vi "Dashboard Main.vi"() -> ()   [LabVIEW 2020]
uses:
  <vilib>/event_ctls.llb/eventvkey.ctl
  <vilib>/Rock Robotics/Network Tables/NT Read Numeric Array.vi
  <vilib>/Rock Robotics/Network Tables/NT Write Boolean Array.vi
  <vilib>/Rock Robotics/WPI/Dashboard/WPI_DashboardLogging Global.vi
panel:
  in  "Camera Settings Right":T1={"Frame Rate"=30, "Compression"=30, "Size"=1, "DB Camera Config"=FALSE} {"Frame Rate" scale=1.0..30.0; "Compression" scale=100.0..-1.0; "Size" items=["640x480", "320x240", "160x120"]}
  in  "Camera Name Right":string(combo)="No Camera Selection"
  out "Camera Perf":string
  in  "Camera Settings":T1={"Frame Rate"=30, "Compression"=30, "Size"=1, "DB Camera Config"=FALSE} {"Frame Rate" scale=1.0..30.0; "Compression" scale=100.0..-1.0; "Size" items=["640x480", "320x240", "160x120"]}
  in  "TCP":refnum<k5>
  in  "Rec Mode":enum32{"Stop", "Record", "Playback"}(radio)
  out "Robot IP":string
  out "Image Message":string="Timeout in Camera Communications"
  in  "Dashboard Tab":T2(tab)
  out "HAD Left Deployment":dbl
  out "HAD Right Deployment":dbl
  out "EXC Right Deployment":dbl
  out "EXC Left Deployment":dbl
  out "Robot Velocity":dbl
  in  "Select Auto":string(combo)="Select Autonomous ..."
  out "NT Connection":bool
  out "MotorChart R":cluster{"Numeric":dbl, "Numeric":dbl}(graph)
  out "MotorChart L":cluster{"Numeric":dbl, "Numeric":dbl}(graph)
  out "MotorSliders R":cluster{"MotorSlide1":dbl, "MotorSlide2":dbl} {"MotorSlide2" scale=-1.0..1.0 scale format="%#_2e"; "MotorSlide1" scale=-1.0..1.0 scale format="%#_2e"}
  out "MotorSliders L":cluster{"MotorSlide1":dbl, "MotorSlide2":dbl} {"MotorSlide2" scale=-1.0..1.0 scale format="%#_2e"; "MotorSlide1" scale=-1.0..1.0 scale format="%#_2e"}
  out "Gyro":dbl(knob) scale=0.0..360.0
  out "JS1 Z":dbl(slide) scale=-1.0..1.0 scale format="%#_2e"
  out "JS1 Graph":cluster{"X":dbl, "Y":dbl}[](graph)
  out "JS1 Buttons":T3
  out "JS2 Z":dbl(slide) scale=-1.0..1.0 scale format="%#_2e"
  out "JS2 Graph":cluster{"X":dbl, "Y":dbl}[](graph)
  out "JS2 Buttons":T3
  out "Mode":T4(ring)=enum."Auto Disabled"
  out "Right Camera Perf":cluster{"Bandwidth (Mbps)":dbl, "FPS":dbl}
  out "Current State":string
  in  "Return EXC":bool
  in  "Approach Berm":bool
  in  "Drive to Dep":bool
  in  "Return Trench":bool
  in  "Auto Traverse":bool
  in  "HAD Deploy":bool
  in  "HAD Deposit":bool
  in  "HAD Retract":bool
  in  "EXC Retract":bool
  in  "EXC Index":bool
  in  "EXC Inch":bool
  in  "EXC Excavate":bool
  in  "EXC Deploy":bool
  in  "Manual Mode":bool
  in  "EXC Power":dbl
  out "HAD Flat Vel":dbl
  out "EXC Bucket Vel":dbl
  out "Current Consumption Over Time":T5(graph)
  out "Front Left Curr":dbl
  out "Front Right Curr":dbl
  out "Rear Left Curr":dbl
  out "Rear Right Curr":dbl
  out "Camera Image Right":T6(plugin-control)
  in  "DB/String 9":string
  in  "DB/String 8":string
  in  "DB/String 7":string
  in  "DB/String 6":string
  in  "DB/String 5":string
  in  "DB/String 4":string
  in  "DB/String 3":string
  in  "DB/String 2":string
  in  "DB/String 1":string
  in  "DB/String 0":string
  in  "DB/Slider 0":dbl(slide) scale=0.0..5.0
  in  "DB/Slider 1":dbl(slide) scale=0.0..5.0
  in  "DB/Slider 2":dbl(slide) scale=0.0..5.0
  in  "DB/Slider 3":dbl(slide) scale=0.0..5.0
  out "DB/LED 3":bool
  out "DB/LED 2":bool
  out "DB/LED 1":bool
  out "DB/LED 0":bool
  in  "DB/Button 3":bool
  in  "DB/Button 2":bool
  in  "DB/Button 1":bool
  in  "DB/Button 0":bool caption="New Name"
  in  "Test Slider":dbl(slide) scale=0.0..100.0 scale format="%#_3g"
  in  "On/Off":bool caption="Solenoid"
  in  "Test Name":u16(ring) items=["Select the test to run..."]
  in  "Test Tree":string(tree)
  in  "Motor":cluster{"Value":dbl, "Enable":bool} {"Value" scale=-1.0..1.0 scale format="%#_3g"}
  out "Progress":T7 {"Test Progress" scale=0.0..100.0}
  in  "Rev/Fwd":cluster{"Forward":bool, "Reverse":bool}
  in  "Test Ring":u16(ring) items=["Monochrome", "Color"]
  in  "CheckList":i32(listbox)
  out "Tree":string(tree)
  out "Camera Image":T6(plugin-control)
  out "Background":bool
  in  "Camera Name":string(combo)="No Camera Selection"
  # "HW"
  # "HW"
  # "Joysticks"
  # "Drive Motors"
  # "Front"
  # "Right"
  # "Left"
  # "Back"
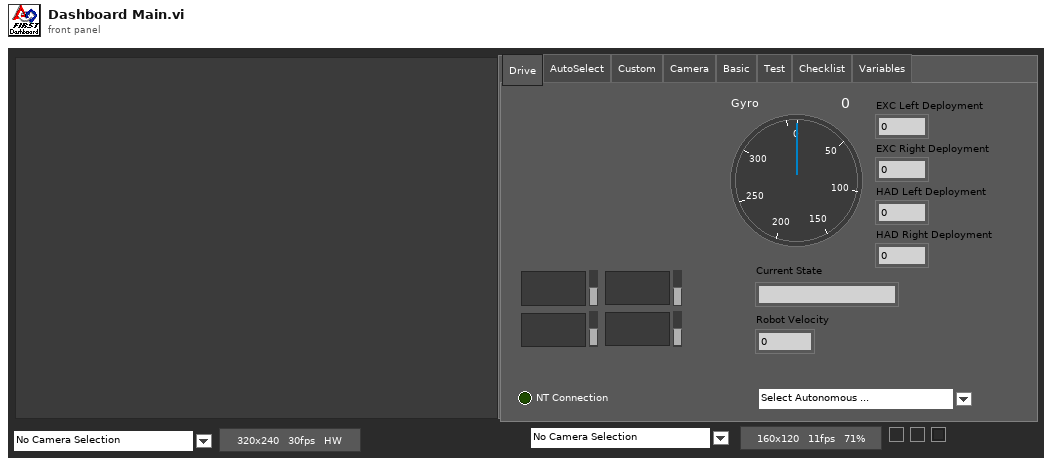
[diagram p1: front panel]
types:
  T1 = cluster{"Frame Rate":i32, "Compression":i32, "Size":u16, "DB Camera Config":bool}
  T2 = enum32{"Drive", "AutoSelect", "Custom", "Camera", "Basic", "Test", "Checklist", "Variables"}
  T3 = cluster{bool, bool, bool, bool, bool, bool, bool, bool, bool, bool, bool, bool}
  T4 = enum8{"Tele-Op Disabled", "Tele-Op Enabled", "Auto Disabled", "Auto Enabled", "Test Disabled", "Test Enabled", "Disconnected", "No Code", "E-Stop"}
  T5 = cluster{"[0]":dbl, "[1]":dbl, "[2]":dbl, "[3]":dbl, "[4]":dbl, "[5]":dbl, "[6]":dbl, "[7]":dbl, "[8]":dbl}
  T6 = typedef "IMAQ Image.ctl" = refnum<image>
  T7 = cluster{"Test Progress":u8, "Test Progress Text":string}
  T8 = cluster{"Save Path":path, "Interval (s)":dbl, "Keep":i32}
  T9 = enum32{"Drive", "Camera", "Basic", "Custom", "Test", "Commands", "Checklist", "Variables"}
  T10 = typedef "Image Type" = u32
  T11 = cluster{"Error Strings":string, "Disable Counts":cluster{u16, u16}, "Rail Faults":cluster{u16, u16, u16}, "Robot IP":string, "DB Mode":u8, "Event Info":cluster{"Name":string, "Type":u8, "Number":u16, "Replay":u8}}
  T12 = cluster{"Storage":cluster{"Disk Free":u64, "RAM Block":u32, "RAM free":u32}, "CPU Utilization":cluster{"CPU % ISR":sgl, "CPU % Time Crit":sgl, "CPU % Timed Str":sgl, "CPU % High":sgl, "CPU % Above":sgl, "CPU % Normal":sgl, "CPU % Low":sgl}, "CAN":cluster{"% Bus Utilization":sgl, "Bus Off Cnt":u32, "TX_FIFO Full Cnt":u32, "Receive Error Cnt":u8, "Transmit Error Cnt":u8}, "HID":cluster{"HID Outputs":u32, "Rumble Low":u16, "Rumble High":u16}[]}
  T13 = cluster{"Status bits":cluster{"Test Mode":bool, "Autonomous":bool, "Enabled":bool, "Code Start":bool, "Brownout":bool, "Reserved 2":bool, "Reserved 3":bool, "E-Stop":bool}, "Code Trace":cluster{"Disabled":bool, "TeleOp":bool, "Auto":bool, "Test":bool}, "Controller Type":enum16{"unknown", "cRIO", "roboRio"}, "Code?":enum16{"unknown", "noCode", "code"}, "Battery V":dbl}
  T14 = cluster{"Control Bits":cluster{"TestMode":bool, "Autonomous":bool, "Enabled":bool, "FMS Present":bool, bool, bool, bool, "E-Stop":bool}, "Team Station ":u8, "Countdown":sgl, "Joystick Values":cluster{"Axes":dbl[], "Buttons":bool[], "POVs":i16[]}[]}
  T15 = cluster{"Axes":dbl[], "Buttons":bool[], "POVs":i16[]}[]
  T16 = cluster{"Axes":dbl[], "Buttons":bool[], "POVs":i16[]}
  T17 = cluster{"Buttons[0]":bool, "Buttons[1]":bool, "Buttons[2]":bool, "Buttons[3]":bool, "Buttons[4]":bool, "Buttons[5]":bool, "Buttons[6]":bool, "Buttons[7]":bool, "Buttons[8]":bool, "Buttons[9]":bool, "Buttons[10]":bool, "Buttons[11]":bool}
  T18 = cluster{"Camera Image":refnum<vi>, "Dashboard Tab":refnum<vi>, "Background":refnum<vi>, "Rec Mode":refnum<vi>, "Test Slider":refnum<vi>, "On/Off ":refnum<vi>, "Test Ring":refnum<vi>, "Rev/Fwd":refnum<vi>, "Test Name":refnum<vi>, "Motor":refnum<vi>, "Progress":refnum<vi>, "CheckList":refnum<vi>, "Tree":refnum<vi>, "Test Tree":refnum<vi>, "Camera Settings":refnum<vi>, "Camera Name":refnum<vi>, "Camera Perf":refnum<vi>, "Camera Settings Right":refnum<vi>, "Camera Name Right":refnum<vi>, "Camera Image Right":refnum<vi>}
  T19 = cluster{"Global Rectangle":i32[], "Contours":cluster{"Contour Type":u32, "ROI Type":u32, "Points":i32[]}[]}
  T20 = cluster{"Camera Name":string, string, "Saved DB Images Info":cluster{"Save Path":path, "Interval (s)":dbl, "Keep":i32}}
  T21 = cluster{"Camera Name Right":string, string, "Saved DB Images Info":cluster{"Save Path":path, "Interval (s)":dbl, "Keep":i32}}
  T22 = cluster{"Operation":enum16{"Update", "Clear"}, "Color Box":u32}[]
  T23 = typedef "eventvkey.ctl" = enum16{"ASCII", "Enter", "Return", "Shift", "Ctrl", "Alt", "Cmd", "Opt", "Caps", "NumLock", "Clear", "Break", "Up", "Down", "Left", "Right", "Insert", "Delete", "Home", "End", "PageUp", "PageDown", "Escape", "Help", "Pause", "ScrollLock", "F1", "F2", "F3", "F4", "F5", "F6", "F7", "F8", "F9", "F10", "F11", "F12", "F13", "F14", "F15", "F16", "F17", "F18", "F19", "F20", "F21", "F22", "F23", "F24", "Play", "VolumeUp", "VolumeDown", "Mute", "Two Byte Char"}
  T24 = cluster{"Image Size":bool, "Image Type":bool, "Pixel Value":bool, "ROI Information":bool, "Zoom Factor":bool}
  T25 = cluster{"Operation":enum16{"Update", "Clear"}, "Color Box":u32}
  T26 = cluster{"Shift":bool, "Ctrl":bool, "Alt":bool, "Cmd":bool, "Opt":bool}
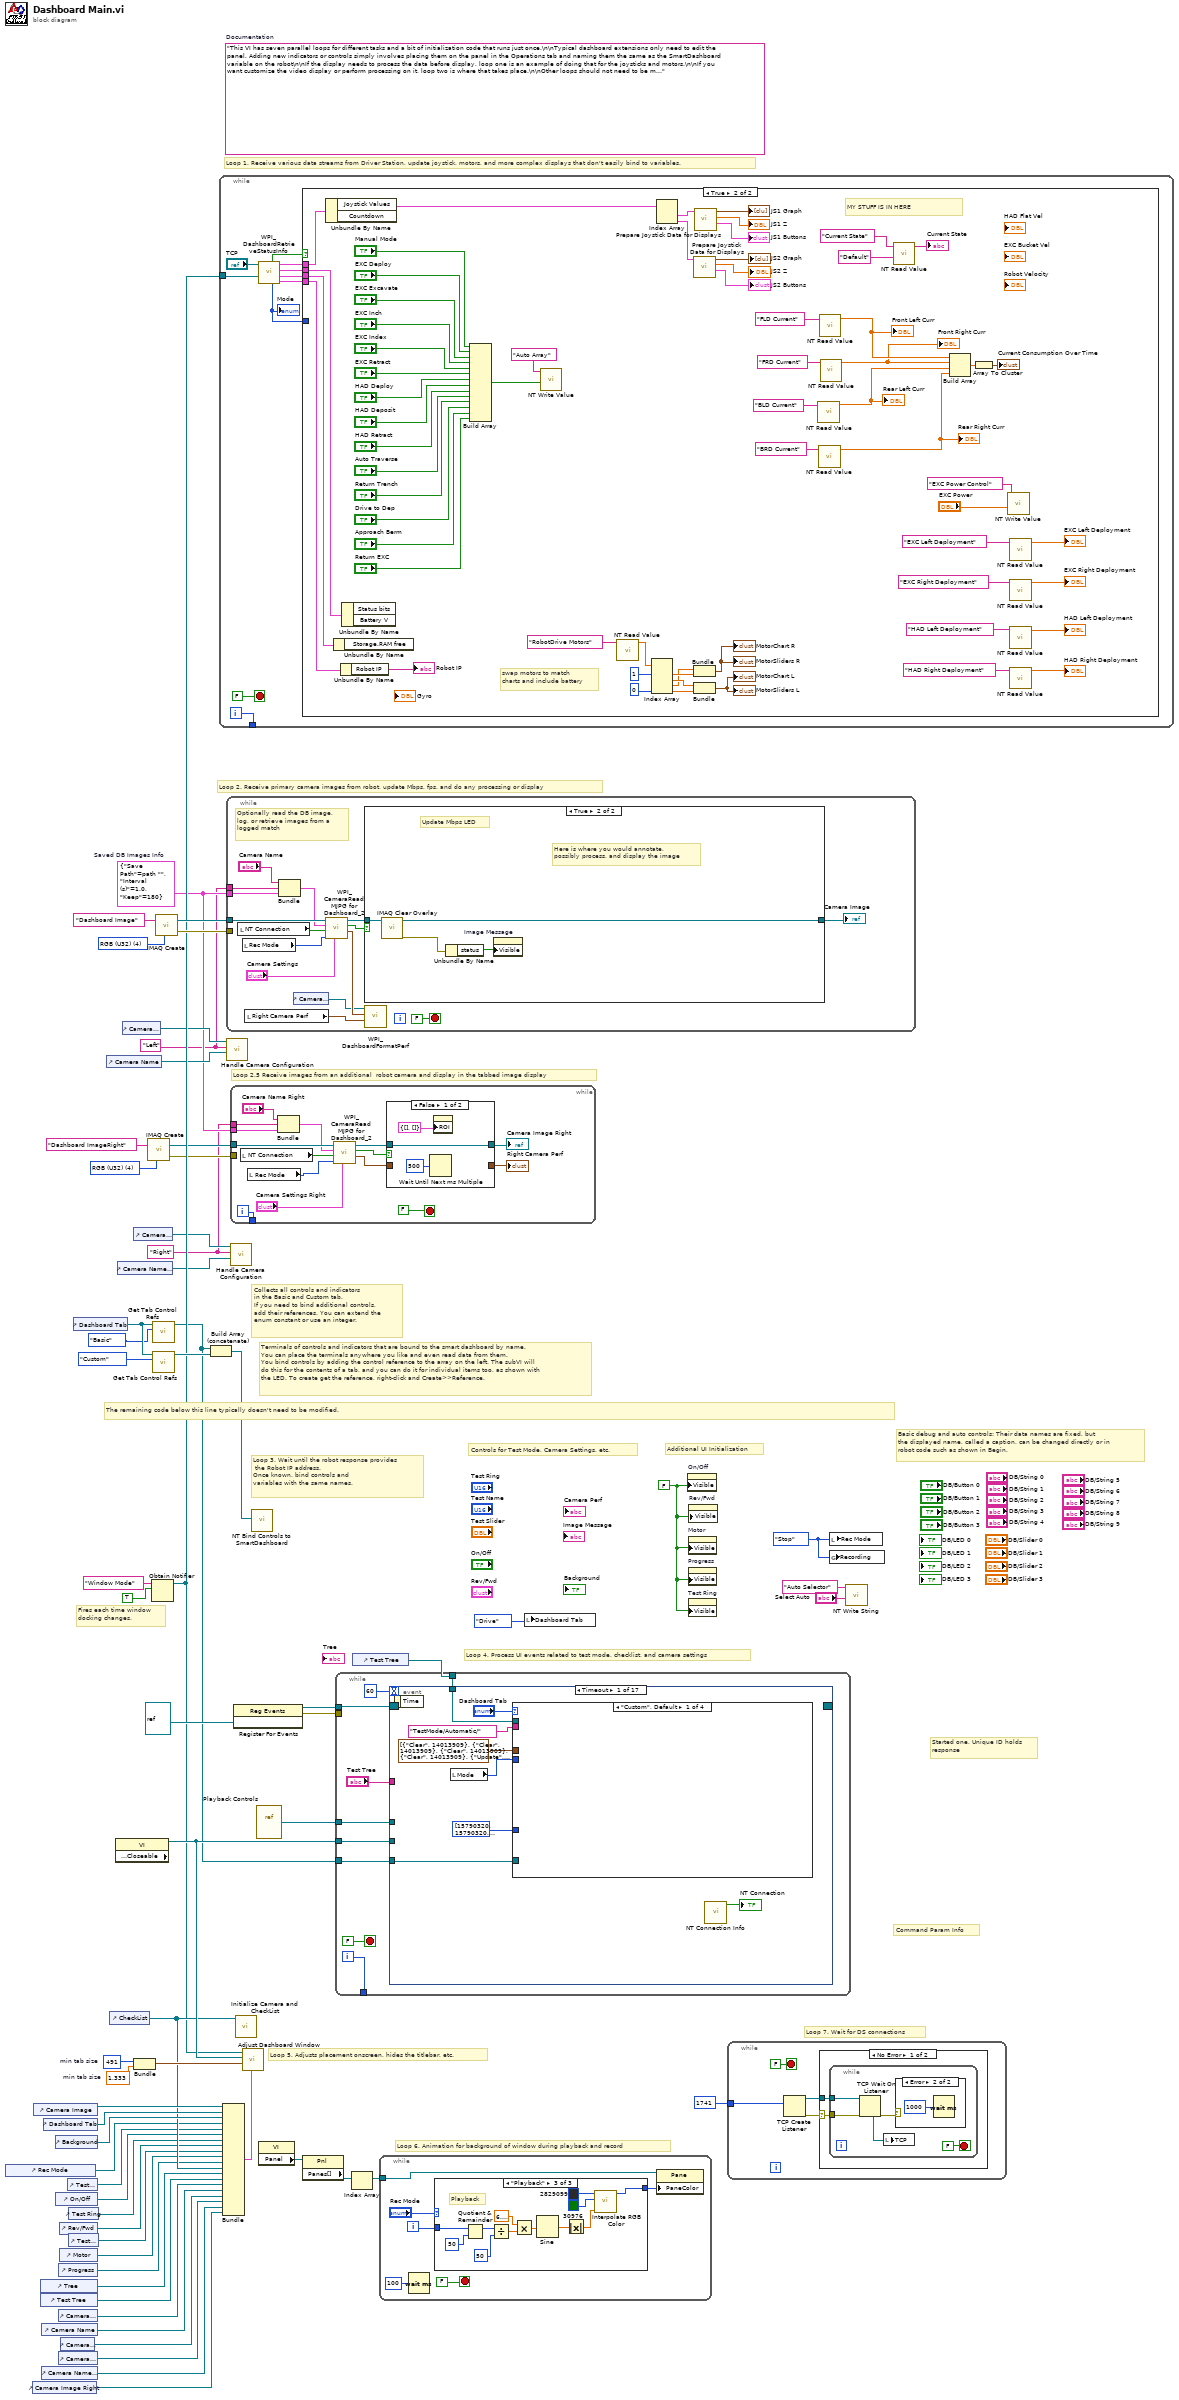
[diagram p0: block diagram]
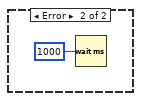
[diagram p4: hidden frame]
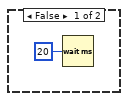
[diagram p5: hidden frame]
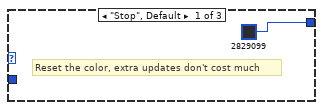
[diagram p6: hidden frame]
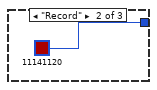
[diagram p7: hidden frame]
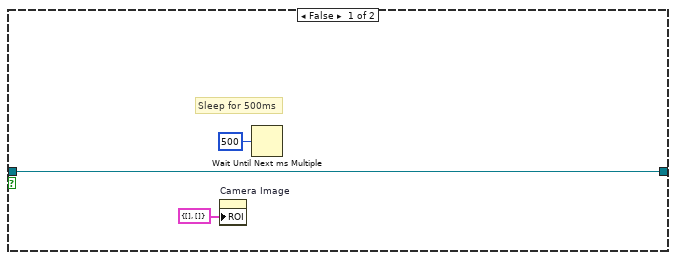
[diagram p8: hidden frame]
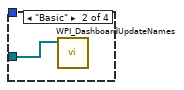
[diagram p9: hidden frame]
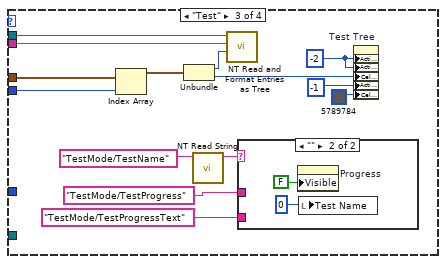
[diagram p10: hidden frame]
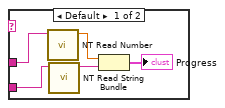
[diagram p11: hidden frame]
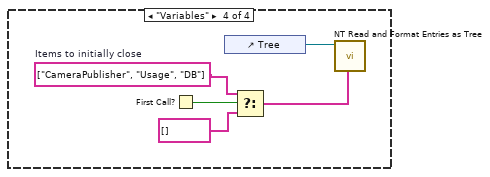
[diagram p12: hidden frame]
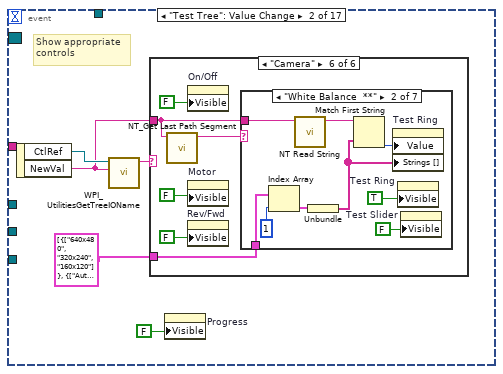
[diagram p13: hidden frame]
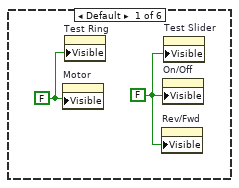
[diagram p14: hidden frame]
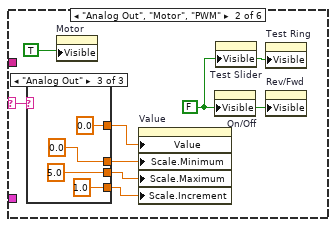
[diagram p15: hidden frame]
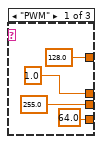
[diagram p16: hidden frame]
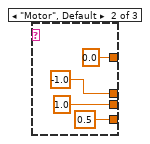
[diagram p17: hidden frame]
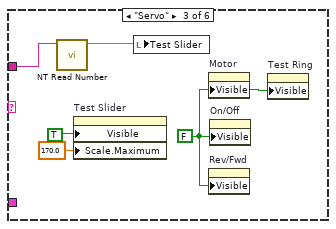
[diagram p18: hidden frame]
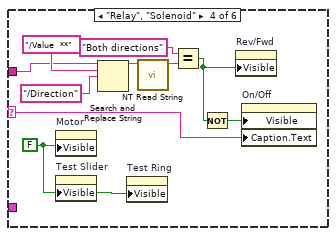
[diagram p19: hidden frame]
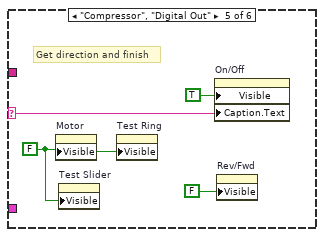
[diagram p20: hidden frame]
diagram:
  w4 = T8 {"Save Path"=path "", "Interval (s)"=1.0, "Keep"=180}  # Saved DB Images Info
  w3 = "Right"
  w2 = "Left"
  w14 = T10 4 items=["Grayscale (U8)", "Grayscale (I16)", "Grayscale (SGL)", "Complex (CSG)", "RGB (U32)", "HSL (U32)", "RGB (U64)"] ("Image Type")
  w42 = 491  # min tab size
  w41 = 1.333  # min tab size
  w49 = enum32{"Stop", "Record", "Playback"}."Stop" ("Rec Mode")
  w26 = FALSE ("Visible")
  (unwired) "This VI has seven parallel loops for different tasks and a bit of initialization code that runs just once.\n\nTypical dashboard extensions only need to edit the panel. Adding new indicators or controls simply involves placing them on the panel in the Operations tab and naming them the same as the SmartDashboard variable on the robot\n\nIf the display needs to process the data before display, loop one is an example of doing that for the joysticks and motors.\n\nIf you want customize the video display or perform processing on it, loop two is where that takes place.\n\nOther loops should not need to be modified. They are pretty standard, and document the task they perform."  # Documentation
  w63 = T10 4 items=["Grayscale (U8)", "Grayscale (I16)", "Grayscale (SGL)", "Complex (CSG)", "RGB (U32)", "HSL (U32)", "RGB (U64)"] ("Image Type")
  # "Loop 2.5 Receive images from an additional  robot camera and display in the tabbed image display"
  # "Command Param Info"
  # "Started one, Unique ID holds\nresponse"
  # "Loop 7. Wait for DS connections"
  # "Basic debug and auto controls: Their data names are fixed, but\nthe displayed name, called a caption, can be changed directly or in\nrobot code such as shown in Begin."
  # "Controls for Test Mode, Camera Settings, etc."
  # "Additional UI Initialization"
  # "Loop 6. Animation for background of window during playback and record"
  # "Fires each time window\ndocking changes."
  # "Collects all controls and indicators\nin the Basic and Custom tab.\nIf you need to bind additional controls,\nadd their references. You can extend the\nenum constant or use an integer."
  # "The remaining code below this line typically doesn't need to be modified."
  # "Loop 4. Process UI events related to test mode, checklist, and camera settings"
  # "Terminals of controls and indicators that are bound to the smart dashboard by name.\nYou can place the terminals anywhere you like and even read data from them.\nYou bind controls by adding the control reference to the array on the left. The subVI will\ndo this for the contents of a tab, and you can do it for individual items too, as shown with\nthe LED. To create get the reference, right-click and Create>>Reference."
  # "Loop 3. Wait until the robot response provides\n the Robot IP address.\nOnce known, bind controls and\nvariables with the same names."
  # "Loop 5. Adjusts placement onscreen, hides the titlebar, etc."
  # "Loop 1. Receive various data streams from Driver Station, update joystick, motors, and more complex displays that don't easily bind to variables."
  # "Loop 2. Receive primary camera images from robot, update Mbps, fps, and do any processing or display"
  n1 = control-ref of="Rec Mode"() -> (w32:refnum<vi>)
  n2 = control-ref of="Camera Image Right"() -> (w7:refnum<vi>)
  n3 = control-ref of="Camera Image"() -> (w44:refnum<vi>)
  n4 = control-ref of="Tree"() -> (w36:refnum<vi>)
  n5 = control-ref of="Test Tree"() -> (w35:refnum<vi>)
  n6 = control-ref of="Camera Name"() -> (w20:refnum<vi>)
  n7 = control-ref of="Camera Name Right"() -> (w8:refnum<vi>)
  n8 = control-ref of="Dashboard Tab"() -> (w43:refnum<vi>)
  n9 = control-ref of="Background"() -> (w39:refnum<vi>)
  n10 = control-ref of="On/Off"() -> (w30:refnum<vi>)
  n11 = control-ref of="Progress"() -> (w27:refnum<vi>)
  n12 = control-ref of="Camera Settings"() -> (w21:refnum<vi>)
  n13 = control-ref of="Camera Settings Right"() -> (w9:refnum<vi>)
  n14 = control-ref of="Rev/Fwd"() -> (w28:refnum<vi>)
  n15 = control-ref of="Motor"() -> (w33:refnum<vi>)
  n16 = control-ref of="Camera Perf"() -> (w19:refnum<vi>)
  n17 = control-ref of="Test Slider"() -> (w31:refnum<vi>)
  n18 = control-ref of="Test Ring"() -> (w29:refnum<vi>)
  n19 = control-ref of="Test Name"() -> (w34:refnum<vi>)
  n20 = control-ref of="Dashboard Tab"() -> (w47:refnum<vi>)
  n21 = control-ref of="Camera Name"() -> (w22:refnum<vi>)
  n22 = control-ref of="CheckList"() -> (w37:refnum<vi>)
  n23 = property class="VI" props=["Front Panel.Closeable"]() -> (reference out=w48:refnum<vi>)  [unwired: 2 in, 2 out]
  n24 = control-ref of="Camera Name Right"() -> (w10:refnum<vi>)
  n25 = control-ref of="Camera Settings"() -> (w23:refnum<vi>)
  n26 = control-ref of="Camera Settings Right"() -> (w11:refnum<vi>)
  n27 = Bundle("min tab size"=w42, "min tab size"=w41) -> (w40:cluster{"min tab size":i32, "min tab size":dbl})  [unwired: 1 in]
  n28 = call "IMAQ Create"("Image Name"="Dashboard ImageRight", "Image Type"=w14) -> ("New Image"=w13:T6, "error out"=w12:errorcluster)  [unwired: 2 in, 1 out]
  n29 = Obtain Notifier(name (unnamed)="Window Mode", notification data type=TRUE) -> (notifier out=w25:refnum<notifier>)  [unwired: 2 in, 2 out]
  n30 = call <vilib>:"Get Tab Control Refs.vi"("Page Index"=T9."Basic" ("Dashboard Tab"), "TabControl in"=w47) -> ("ControlsOnPage"=w18:refnum<vi>[])  [unwired: 9 in]
  n31 = call <vilib>:"Get Tab Control Refs.vi"("Page Index"=T9."Custom" ("Dashboard Tab"), "TabControl in"=w47) -> ("ControlsOnPage"=w46:refnum<vi>[])  [unwired: 9 in]
  n32 = call "IMAQ Create"("Image Name"="Dashboard Image", "Image Type"=w63) -> ("New Image"=w61:T6, "error out"=w60:errorcluster)  [unwired: 2 in, 1 out]
  n33 = Build Array (concatenate)(w18, w46) -> (w45:refnum<vi>[])
  n34 = while {
    tunnel: [w72] -> _
    tunnel: w25 -> [w64]
    i -> [w72]
    stop <- FALSE stop-if-true
    n35 = call <vilib>:"WPI_DashboardRetrieveStatusInfo.vi"("Window Mode Notifier"=w64, "TCP Cnx"="TCP") -> ("Power and Errors"=w67:T11, "Robot Metrics"=w70:T12, "Status Info"=w71:T13, "Control Info"=w68:T14, "Robot Mode"=w66:T4, "Process?"=w69:bool)  [unwired: 4 in]
    "Mode" <- w66
    n36 = case shown="True" w69 {
      tunnel: w71 -> [_ w137]
      tunnel: w70 -> [_ w136]
      tunnel: w68 -> [_ w135]
      tunnel: w67 -> [_ w134]
      tunnel: w66 -> [_ _]
      frame False {
        n37 = Wait (ms)(milliseconds to wait=u32 20) -> ()  [unwired: 1 out]
      }
      frame True {
        # "MY STUFF IS IN HERE"
        # "swap motors to match\ncharts and include battery"
        n38 = Unbundle By Name(w135) -> ("Joystick Values"=w125:T15)  [unwired: 1 out]
        n39 = Unbundle By Name(w136) -> ()  [unwired: 1 out]
        n40 = Unbundle By Name(w134) -> ("Robot IP"=→"Robot IP":string)
        n41 = Unbundle By Name(w137) -> ()  [unwired: 2 out]
        n42 = Build Array("Manual Mode", "EXC Deploy", "EXC Excavate", "EXC Inch", "EXC Index", "EXC Retract", "HAD Deploy", "HAD Deposit", "HAD Retract", "Auto Traverse", "Return Trench", "Drive to Dep", "Approach Berm", "Return EXC") -> (w75:bool[])
        n43 = call-poly <vilib>:"NT Write Value.vi"("value"=w75, "name"="Auto Array") -> ()  [unwired: 9 in, 1 out]
        n44 = call-poly <vilib>:"NT Read Value.vi"("name"="RobotDrive Motors" ("Name")) -> ("value"=w115:dbl[])  [unwired: 8 in, 2 out]
        n45 = Index Array(array=w115, index #1=1, index #4=0) -> (element #1=w129:dbl, element #2=w130:dbl, element #3=w128:dbl, element #4=w133:dbl)  [unwired: 2 in]
        n46 = Index Array(array=w125) -> (element #1=w124:T16, element #2=w120:T16)  [unwired: 2 in]
        n47 = call "Prepare Joystick Data for Displays.vi"("Joystick Values"=w120) -> ("Buttons"=→"JS2 Buttons":T17, "Z Axis"=→"JS2 Z":dbl, "Cartesian Data"=→"JS2 Graph":cluster{"X axis":dbl, "X axis":dbl}[])  [unwired: 8 in]
        n48 = Bundle("Numeric"=w128, "Numeric"=w129) -> (→"MotorChart R" →"MotorSliders R":cluster{"Numeric":dbl, "Numeric":dbl})  [unwired: 1 in]
        n49 = Bundle("Numeric"=w130, "Numeric"=w133) -> (→"MotorChart L" →"MotorSliders L":cluster{"Numeric":dbl, "Numeric":dbl})  [unwired: 1 in]
        n50 = call "Prepare Joystick Data for Displays.vi"("Joystick Values"=w124) -> ("Buttons"=→"JS1 Buttons":T17, "Z Axis"=→"JS1 Z":dbl, "Cartesian Data"=→"JS1 Graph":cluster{"X axis":dbl, "X axis":dbl}[])  [unwired: 8 in]
        n51 = call-poly <vilib>:"NT Read Value.vi"("name"="BLD Current") -> ("value"=w100:dbl)  [unwired: 8 in, 2 out]
        "Rear Left Curr" <- w100
        n52 = call-poly <vilib>:"NT Read Value.vi"("name"="BRD Current") -> ("value"=w101:dbl)  [unwired: 8 in, 2 out]
        "Rear Right Curr" <- w101
        n53 = call-poly <vilib>:"NT Read Value.vi"("name"="FLD Current") -> ("value"=w103:dbl)  [unwired: 8 in, 2 out]
        "Front Left Curr" <- w103
        n54 = call-poly <vilib>:"NT Read Value.vi"("name"="FRD Current") -> ("value"=w102:dbl)  [unwired: 8 in, 2 out]
        "Front Right Curr" <- w102
        n55 = call-poly <vilib>:"NT Read Value.vi"("default value"="Default", "name"="Current State") -> ("value"=→"Current State":string)  [unwired: 7 in, 2 out]
        n56 = Build Array(w103, w102, w100, w101) -> (w105:dbl[])
        n57 = Array To Cluster(array=w105) -> (cluster=→"Current Consumption Over Time":T5)
        n58 = call-poly <vilib>:"NT Write Value.vi"("value"="EXC Power", "name"="EXC Power Control") -> ()  [unwired: 9 in, 1 out]
        n59 = call-poly <vilib>:"NT Read Value.vi"("name"="EXC Left Deployment") -> ("value"=→"EXC Left Deployment":dbl)  [unwired: 8 in, 2 out]
        n60 = call-poly <vilib>:"NT Read Value.vi"("name"="EXC Right Deployment") -> ("value"=→"EXC Right Deployment":dbl)  [unwired: 8 in, 2 out]
        n61 = call-poly <vilib>:"NT Read Value.vi"("name"="HAD Left Deployment") -> ("value"=→"HAD Left Deployment":dbl)  [unwired: 8 in, 2 out]
        n62 = call-poly <vilib>:"NT Read Value.vi"("name"="HAD Right Deployment") -> ("value"=→"HAD Right Deployment":dbl)  [unwired: 8 in, 2 out]
      }
    }
  }
  n63 = Bundle("Camera Image"=w44, "Dashboard Tab"=w43, "Background"=w39, "Rec Mode"=w32, "Test Slider"=w31, "On/Off"=w30, "Test Ring"=w29, "Rev/Fwd"=w28, "Test Name"=w34, "Motor"=w33, "Progress"=w27, "CheckList"=w37, "Tree"=w36, "Test Tree"=w35, "Camera Settings"=w21, "Camera Name"=w20, "Camera Perf"=w19, "Camera Settings Right"=w9, "Camera Name Right"=w8, "Camera Image Right"=w7) -> (w38:T18)  [unwired: 1 in]
  n64 = call "Handle Camera Configuration.vi"("CameraNameRef"=w22, "Display Name"=w2, "ClusterRef"=w23) -> ()  [unwired: 9 in]
  n65 = while {
    tunnel: w61 -> [w151]
    tunnel: w60 -> [_]
    tunnel: w4 -> [w144]
    tunnel: w2 -> [w141]
    stop <- FALSE stop-if-true
    # "Optionally read the DB image,\nlog, or retrieve images from a\nlogged match"
    n66 = local read "NT Connection"() -> (w145:bool)
    n67 = local read "Rec Mode"() -> (w148:enum32{"Stop", "Record", "Playback"})
    n68 = local read "Right Camera Perf"() -> (w139:cluster{"Bandwidth (Mbps)":dbl, "FPS":dbl})
    n69 = Bundle("Camera Name"="Camera Name", w141, "Saved DB Images Info"=w144) -> (w143:T20)  [unwired: 1 in]
    n70 = control-ref of="Camera Perf"() -> (w138:refnum<vi>)
    n71 = call <vilib>:"WPI_CameraRead MJPG for Dashboard_2.vi"("Camera Settings"="Camera Settings", "Rec Mode"=w148, "NT Connection"=w145, "Capture Info"=w143, "Image in"=w151) -> ("perf info"=w140:cluster{"Bandwidth (Mbps)":dbl, "fps":dbl}, "Active"=w149:bool, "Image\\ out"=w150:T6)  [unwired: 4 in]
    n72 = case shown="True" w149 {
      tunnel: w150 -> [w154 w157]
      tunnel: [w154 w156] -> w146
      frame False {
        # "Sleep for 500ms"
        n73 = property on="Camera Image" class="ImageControl"("ROI"=T19 {"Global Rectangle"=[], "Contours"=[]}) -> ()  [unwired: 2 in, 2 out]
        n74 = Wait Until Next ms Multiple(millisecond multiple=u32 500) -> ()  [unwired: 1 out]
      }
      frame True {
        # "Here is where you would annotate,\npossibly process, and display the image"
        # "Update Mbps LED"
        n75 = call "IMAQ Clear Overlay"("Image"=w157) -> ("error out"=w158:errorcluster, "Image Out"=w156:T6)  [unwired: 2 in, 7 out]
        n76 = Unbundle By Name(w158) -> ("status"=w159:bool)
        n77 = property on="Image Message" class="Str"("Visible"=w159) -> ()  [unwired: 2 in, 2 out]
      }
    }
    "Camera Image" <- w146
    n78 = call <vilib>:"WPI_DashboardFormatPerf.vi"("Right Camera Perf"=w139, "Performance"=w140, "String in"=w138) -> ()  [unwired: 9 in]
  }
  n79 = call "Handle Camera Configuration.vi"("CameraNameRef"=w10, "Display Name"=w3, "ClusterRef"=w11) -> ()  [unwired: 9 in]
  n80 = while {
    tunnel: w13 -> [w174]
    tunnel: w12 -> [_]
    tunnel: [w169] -> _
    tunnel: w4 -> [w165]
    tunnel: w3 -> [w162]
    i -> [w169]
    stop <- FALSE stop-if-true
    n81 = local read "NT Connection"() -> (w166:bool)
    n82 = local read "Rec Mode"() -> (w173:enum32{"Stop", "Record", "Playback"})
    n83 = Bundle("Camera Name Right"="Camera Name Right", w162, "Saved DB Images Info"=w165) -> (w164:T21)  [unwired: 1 in]
    n84 = call <vilib>:"WPI_CameraRead MJPG for Dashboard_2.vi"("Camera Settings"="Camera Settings Right", "Rec Mode"=w173, "NT Connection"=w166, "Capture Info"=w164, "Image in"=w174) -> ("perf info"=w160:cluster{"Bandwidth (Mbps)":dbl, "fps":dbl}, "Active"=w168:bool, "Image\\ out"=w171:T6)  [unwired: 4 in]
    n85 = case shown="False" w168 {
      tunnel: w171 -> [w176 w179]
      tunnel: [w176 w179] -> w167
      tunnel: [_ w178] -> w161
      tunnel: w160 -> [_ w178]
      frame False {
        n86 = Wait Until Next ms Multiple(millisecond multiple=u32 500) -> ()  [unwired: 1 out]
        n87 = property on="Camera Image Right" class="ImageControl"("ROI"=T19 {"Global Rectangle"=[], "Contours"=[]}) -> ()  [unwired: 2 in, 2 out]
      }
      frame True {
      }
    }
    "Camera Image Right" <- w167
    "Right Camera Perf" <- w161
  }
  n88 = register-events(refnum<vi> refnum) -> (reference out=w52:refnum<event-registration>, error out=w51:errorcluster)  [unwired: 2 in]
  n89 = call "Initialize Camera and CheckList.vi"("ListBox in"=w37) -> ()  [unwired: 11 in]
  n90 = call "Adjust Dashboard Window.vi"("Sizing Refnums"=w38, "Size Constraints"=w40, "VI"=w48, "WIn Mode"=w25) -> ()  [unwired: 8 in]
  n91 = call <vilib>:"NT Bind Controls to SmartDashboard.vi"("Bound Control Refs"=w45) -> ()  [unwired: 11 in]
  n92 = vi-ref "Playback Controls.vi"() -> (w53:refnum<vi>)
  n93 = property class="VI"() -> ("Panel"=w55:refnum<vi>)  [unwired: 2 in, 2 out]
  n94 = property class="Pnl"(reference=w55) -> ("Panes[]"=w56:refnum<vi>[])  [unwired: 1 in, 2 out]
  n95 = Index Array(array=w56) -> (element=w54:refnum<vi>)  [unwired: 1 in]
  n96 = control-ref of="Test Tree"() -> (w57:refnum<vi>)
  n97 = while {
    tunnel: [w185] -> _
    tunnel: w57 -> [w184]
    tunnel: w53 -> [w183]
    tunnel: w52 -> [w182]
    tunnel: w51 -> [_]
    tunnel: w48 -> [w181]
    tunnel: w18 -> [w180]
    i -> [w185]
    stop <- FALSE stop-if-true
    n98 = event shown="[0] Timeout" {
      selector: w182 -> [_ _ _ _ _ _ _ _ _ _ _ _ _ _ _ _ _]
      dyn-events: [_ _ _ _ _ _ _ _ _ _ _ _ _ w390 _ _ _] -> _
      timeout: u32 60 ("milliseconds to wait") -> [_ _ _ _ _ _ _ _ _ _ _ _ _ _ _ _ _]
      tunnel: w184 -> [w195 _ _ _ _ _ _ _ _ _ _ _ _ _ _ _ _]
      tunnel: "Test Tree" -> [_ _ _ _ _ _ _ _ w363 w370 w371 w374 w381 _ _ _ _]
      tunnel: w183 -> [_ _ _ _ _ _ _ _ _ _ _ _ _ w392 _ w407 _]
      tunnel: w181 -> [_ _ _ _ _ _ _ _ _ _ _ _ _ w388 _ _ _]
      tunnel: w180 -> [w190 _ _ _ _ _ _ _ _ _ _ _ _ _ _ _ _]
      event Timeout {
        n99 = event-data() -> ()  [unwired: 1 in, 1 out]
        n100 = local read "Mode"() -> (w193:T4)
        n101 = case shown="\"Custom\", Default" "Dashboard Tab" {
          tunnel: w195 -> [_ _ w211 _]
          tunnel: "TestMode/Automatic/" ("Name Pattern") -> [_ _ w210 _]
          tunnel: T22 [{"Operation"=enum."Clear", "Color Box"=14013909}, {"Operation"=enum."Clear", "Color Box"=14013909}, {"Operation"=enum."Clear", "Color Box"=14013909}, {"Operation"=enum."Clear", "Color Box"=14013909}, {"Operation"=enum."Update", "Color Box"=14013909}, {"Operation"=enum."Update", "Color Box"=16777215}, {"Operation"=enum."Clear", "Color Box"=14013909}, {"Operation"=enum."Clear", "Color Box"=14013909}, {"Operation"=enum."Clear", "Color Box"=14013909}] -> [_ _ w203 _]
          tunnel: w193 -> [_ _ w202 _]
          tunnel: u32[] [15790320, 15790320, 15790320, 15790320, 16777215, 16777215, 15790320, 15790320, 15790320] -> [_ _ _ _]
          tunnel: w190 -> [_ w197 _ _]
          frame "Custom", Default {
          }
          frame "Basic" {
            n102 = call <vilib>:"WPI_DashboardUpdateNames.vi"("Controls on Tab"=w197) -> ()  [unwired: 11 in]
          }
          frame "Test" {
            w209 = -2 ("Active Item:Row Number")
            n103 = Index Array(array=w203, index=w202) -> (element=w204:T25)
            n104 = Unbundle(w204) -> ("Operation"=w205:enum16{"Update", "Clear"}, "Color Box"=w206:u32)
            n105 = call <vilib>:"NT Read String.vi"("name"="TestMode/TestName" ("Name")) -> ("value"=w200:string)  [unwired: 8 in, 2 out]
            n106 = call <vilib>:"NT Read and Format Entries as Tree.vi"("Operation"=w205, "Name Pattern"=w210, "Tree Refnum"=w211) -> ()  [unwired: 7 in, 2 out]
            n107 = case shown="\"\"" w200 {
              tunnel: "TestMode/TestProgress" ("Name") -> [w213 _]
              tunnel: "TestMode/TestProgressText" ("Name") -> [w212 _]
              frame Default {
                n108 = call <vilib>:"NT Read Number.vi"("name"=w213) -> ("value"=w214:dbl)  [unwired: 8 in, 2 out]
                n109 = call <vilib>:"NT Read String.vi"("name"=w212) -> ("value"=w215:string)  [unwired: 8 in, 2 out]
                n110 = Bundle("value"=w214, "value"=w215) -> (→"Progress":cluster{"value":dbl, "value":string})  [unwired: 1 in]
              }
              frame "" {
                n111 = property on="Progress" class="Clust (strict)"("Visible"=FALSE) -> ()  [unwired: 2 in, 2 out]
                n112 = local write "Test Name"(u16 0) -> ()
              }
            }
            n113 = property on="Test Tree" class="Tree (strict)"("Active Item Row Number"=w209, "ActiveColNum"=w209, "CellBG"=w206, "Active Item Row Number"=-1 ("Active Item:Row Number"), "CellBG"=u32 5789784 ("Color Box")) -> ()  [unwired: 2 in, 2 out]
          }
          frame "Variables" {
            w221 = string[] ["CameraPublisher", "Usage", "DB"]  # Items to initially close
            n114 = First Call?() -> (First Call?: T/F=w222:bool)
            n115 = control-ref of="Tree"() -> (w223:refnum<vi>)
            n116 = Select(t=w221, s=w222, f=string[] []) -> (s? t:f=w219:string[])
            n117 = call <vilib>:"NT Read and Format Entries as Tree.vi"("Tags to  Close"=w219, "Tree Refnum"=w223) -> ()  [unwired: 8 in, 2 out]
          }
        }
        n118 = call <vilib>:"NT Connection Info.vi"() -> ("Connected"=→"NT Connection":bool)  [unwired: 11 in]
      }
      event "Test Tree": Value Change {
        # "Show appropriate\ncontrols"
        n119 = event-data() -> ("CtlRef"=w227:refnum<vi>, "NewVal"=w225:string)  [unwired: 1 in]
        n120 = call <vilib>:"WPI_UtilitiesGetTreeIOName.vi"("NewVal"=w225, "TreeControl in"=w227) -> ("I/O Name"=w228:string)  [unwired: 9 in]
        n121 = case shown="\"Camera\"" w228 {
          selector: w228 -> [_ w235 _ w257 w266 _]
          tunnel: w225 -> [_ _ w254 w256 _ w273]
          tunnel: cluster{string[]}[] [{["640x480", "320x240", "160x120"]}, {["Auto", "Fixed indoor", "Fixed outdoor 1", "Fixed outdoor 2", "Fixed fluorescent 1", "Fixed fluorescent 2", "Hold current"]}, {["Auto", "Flicker-free 50 Hz", "Flicker-free 60 Hz", "Hold current"]}, {["None", "Prioritize frame rate", "Prioritize image quality"]}, {["Monochrome", "Color"]}] -> [_ _ _ _ _ w272]
          frame Default {
            w230 = FALSE ("Visible")
            w229 = FALSE ("Visible")
            n122 = property on="Motor" class="Clust (strict)"("Visible"=w229) -> ()  [unwired: 2 in, 2 out]
            n123 = property on="Test Ring" class="Ring (strict)"("Visible"=w229) -> ()  [unwired: 2 in, 2 out]
            n124 = property on="Rev/Fwd" class="Clust (strict)"("Visible"=w230) -> ()  [unwired: 2 in, 2 out]
            n125 = property on="On/Off" class="Bool (strict)"("Visible"=w230) -> ()  [unwired: 2 in, 2 out]
            n126 = property on="Test Slider" class="Slide (strict)"("Visible"=w230) -> ()  [unwired: 2 in, 2 out]
          }
          frame "Analog Out", "Motor", "PWM" {
            w236 = FALSE ("Visible")
            n127 = case shown="\"Analog Out\"" w235 {
              tunnel: [1.0 ("Value") -1.0 ("Value") 0.0 ("Value")] -> w234
              tunnel: [255.0 ("Value") 1.0 ("Value") 5.0 ("Value")] -> w233
              tunnel: [128.0 ("Value") 0.0 ("Value") 0.0 ("Value")] -> w232
              tunnel: [64.0 ("Value") 0.5 ("Value") 1.0 ("Value")] -> w231
              frame "PWM" {
              }
              frame "Motor", Default {
              }
              frame "Analog Out" {
              }
            }
            n128 = property on="Motor" class="Clust (strict)"("Visible"=TRUE) -> ()  [unwired: 2 in, 2 out]
            n129 = property on="Value" class="Slide (strict)"("Value"=w232, "Scale.Minimum"=w234, "Scale.Maximum"=w233, "Scale.Increment"=w231) -> ()  [unwired: 2 in, 2 out]
            n130 = property on="On/Off" class="Bool (strict)"("Visible"=w236) -> ()  [unwired: 2 in, 2 out]
            n131 = property on="Test Slider" class="Slide (strict)"("Visible"=w236) -> ()  [unwired: 2 in, 2 out]
            n132 = property on="Test Ring" class="Ring (strict)"("Visible"=w236) -> ()  [unwired: 2 in, 2 out]
            n133 = property on="Rev/Fwd" class="Clust (strict)"("Visible"=w236) -> ()  [unwired: 2 in, 2 out]
          }
          frame "Servo" {
            w252 = FALSE ("Visible")
            n134 = call <vilib>:"NT Read Number.vi"("name"=w254) -> ("value"=w253:dbl)  [unwired: 8 in, 2 out]
            n135 = property on="Test Slider" class="Slide (strict)"("Visible"=TRUE, "Scale.Maximum"=170.0 ("Scale.Range:Maximum")) -> ()  [unwired: 2 in, 2 out]
            n136 = local write "Test Slider"(w253) -> ()
            n137 = property on="Motor" class="Clust (strict)"("Visible"=w252) -> ()  [unwired: 2 in, 2 out]
            n138 = property on="Rev/Fwd" class="Clust (strict)"("Visible"=w252) -> ()  [unwired: 2 in, 2 out]
            n139 = property on="On/Off" class="Bool (strict)"("Visible"=w252) -> ()  [unwired: 2 in, 2 out]
            n140 = property on="Test Ring" class="Ring (strict)"("Visible"=w252) -> ()  [unwired: 2 in, 2 out]
          }
          frame "Relay", "Solenoid" {
            w255 = FALSE ("Visible")
            n141 = property on="Motor" class="Clust (strict)"("Visible"=w255) -> ()  [unwired: 2 in, 2 out]
            n142 = property on="Test Slider" class="Slide (strict)"("Visible"=w255) -> ()  [unwired: 2 in, 2 out]
            n143 = Search and Replace String(input string=w256, search string="/Value  **", replace string="/Direction") -> (result string=w262:string)  [unwired: 5 in, 3 out]
            n144 = property on="Test Ring" class="Ring (strict)"("Visible"=w255) -> ()  [unwired: 2 in, 2 out]
            n145 = call <vilib>:"NT Read String.vi"("name"=w262) -> ("value"=w260:string)  [unwired: 8 in, 2 out]
            n146 = Equal?(x="Both directions", y=w260) -> (x = y?=w258:bool)
            n147 = Not(x=w258) -> (.not. x?=w259:bool)
            n148 = property on="Rev/Fwd" class="Clust (strict)"("Visible"=w258) -> ()  [unwired: 2 in, 2 out]
            n149 = property on="On/Off" class="Bool (strict)"("Visible"=w259, "Caption.Text"=w257) -> ()  [unwired: 2 in, 2 out]
          }
          frame "Compressor", "Digital Out" {
            w265 = FALSE ("Visible")
            # "Get direction and finish"
            n150 = property on="Motor" class="Clust (strict)"("Visible"=w265) -> ()  [unwired: 2 in, 2 out]
            n151 = property on="Test Slider" class="Slide (strict)"("Visible"=w265) -> ()  [unwired: 2 in, 2 out]
            n152 = property on="Test Ring" class="Ring (strict)"("Visible"=w265) -> ()  [unwired: 2 in, 2 out]
            n153 = property on="On/Off" class="Bool (strict)"("Visible"=TRUE, "Caption.Text"=w266) -> ()  [unwired: 2 in, 2 out]
            n154 = property on="Rev/Fwd" class="Clust (strict)"("Visible"=FALSE) -> ()  [unwired: 2 in, 2 out]
          }
          frame "Camera" {
            n155 = call <vilib>:"NT_Get Last Path Segment.vi"("String in"=w273) -> ("String out"=w274:string)  [unwired: 10 in]
            n156 = property on="On/Off" class="Bool (strict)"("Visible"=FALSE) -> ()  [unwired: 2 in, 2 out]
            n157 = property on="Motor" class="Clust (strict)"("Visible"=FALSE) -> ()  [unwired: 2 in, 2 out]
            n158 = property on="Rev/Fwd" class="Clust (strict)"("Visible"=FALSE) -> ()  [unwired: 2 in, 2 out]
            n159 = case shown="\"White Balance  **\"" w274 {
              tunnel: w273 -> [w280 w289 w298 w307 w316 _ w322]
              tunnel: w272 -> [w278 w286 w295 w304 w313 _ _]
              frame "Size  **" {
                n160 = Index Array(array=w278) -> (element=w277:cluster{string[]})  [unwired: 1 in]
                n161 = call <vilib>:"NT Read String.vi"("name"=w280) -> ("value"=w279:string)  [unwired: 8 in, 2 out]
                n162 = Unbundle(w277) -> (w275:string[])
                n163 = Match First String(2:w275, 3:w279) -> (0:w276:i32)  [unwired: 1 out]
                n164 = property on="Test Ring" class="Ring (strict)"("Value"=w276, "Strings []"=w275) -> ()  [unwired: 2 in, 2 out]
                n165 = property on="Test Ring" class="Ring (strict)"("Visible"=TRUE) -> ()  [unwired: 2 in, 2 out]
                n166 = property on="Test Slider" class="Slide (strict)"("Visible"=FALSE) -> ()  [unwired: 2 in, 2 out]
              }
              frame "White Balance  **" {
                n167 = Index Array(array=w286, index=1) -> (element=w287:cluster{string[]})
                n168 = call <vilib>:"NT Read String.vi"("name"=w289) -> ("value"=w288:string)  [unwired: 8 in, 2 out]
                n169 = Unbundle(w287) -> (w284:string[])
                n170 = Match First String(2:w284, 3:w288) -> (0:w283:i32)  [unwired: 1 out]
                n171 = property on="Test Ring" class="Ring (strict)"("Value"=w283, "Strings []"=w284) -> ()  [unwired: 2 in, 2 out]
                n172 = property on="Test Ring" class="Ring (strict)"("Visible"=TRUE) -> ()  [unwired: 2 in, 2 out]
                n173 = property on="Test Slider" class="Slide (strict)"("Visible"=FALSE) -> ()  [unwired: 2 in, 2 out]
              }
              frame "Exposure  **" {
                n174 = Index Array(array=w295, index=2) -> (element=w296:cluster{string[]})
                n175 = call <vilib>:"NT Read String.vi"("name"=w298) -> ("value"=w297:string)  [unwired: 8 in, 2 out]
                n176 = Unbundle(w296) -> (w292:string[])
                n177 = Match First String(2:w292, 3:w297) -> (0:w293:i32)  [unwired: 1 out]
                n178 = property on="Test Ring" class="Ring (strict)"("Value"=w293, "Strings []"=w292) -> ()  [unwired: 2 in, 2 out]
                n179 = property on="Test Ring" class="Ring (strict)"("Visible"=TRUE) -> ()  [unwired: 2 in, 2 out]
                n180 = property on="Test Slider" class="Slide (strict)"("Visible"=FALSE) -> ()  [unwired: 2 in, 2 out]
              }
              frame "Exposure Priority  **" {
                n181 = Index Array(array=w304, index=3) -> (element=w305:cluster{string[]})
                n182 = call <vilib>:"NT Read String.vi"("name"=w307) -> ("value"=w306:string)  [unwired: 8 in, 2 out]
                n183 = Unbundle(w305) -> (w301:string[])
                n184 = Match First String(2:w301, 3:w306) -> (0:w302:i32)  [unwired: 1 out]
                n185 = property on="Test Ring" class="Ring (strict)"("Value"=w302, "Strings []"=w301) -> ()  [unwired: 2 in, 2 out]
                n186 = property on="Test Ring" class="Ring (strict)"("Visible"=TRUE) -> ()  [unwired: 2 in, 2 out]
                n187 = property on="Test Slider" class="Slide (strict)"("Visible"=FALSE) -> ()  [unwired: 2 in, 2 out]
              }
              frame "Color Enable  **" {
                n188 = Index Array(array=w313, index=4) -> (element=w314:cluster{string[]})
                n189 = call <vilib>:"NT Read String.vi"("name"=w316) -> ("value"=w315:string)  [unwired: 8 in, 2 out]
                n190 = Unbundle(w314) -> (w310:string[])
                n191 = Match First String(2:w310, 3:w315) -> (0:w311:i32)  [unwired: 1 out]
                n192 = property on="Test Ring" class="Ring (strict)"("Value"=w311, "Strings []"=w310) -> ()  [unwired: 2 in, 2 out]
                n193 = property on="Test Ring" class="Ring (strict)"("Visible"=TRUE) -> ()  [unwired: 2 in, 2 out]
                n194 = property on="Test Slider" class="Slide (strict)"("Visible"=FALSE) -> ()  [unwired: 2 in, 2 out]
              }
              frame Default {
                n195 = property on="Test Ring" class="Ring (strict)"("Visible"=FALSE) -> ()  [unwired: 2 in, 2 out]
                n196 = property on="Test Slider" class="Slide (strict)"("Visible"=FALSE) -> ()  [unwired: 2 in, 2 out]
              }
              frame "Brightness  **", "Color Level  **", "Compression  **", "FPS  **", "Sharpness  **" {
                n197 = call <vilib>:"NT Read Number.vi"("name"=w322) -> ("value"=w321:dbl)  [unwired: 8 in, 2 out]
                n198 = local write "Test Slider"(w321) -> ()
                n199 = property on="Test Slider" class="Slide (strict)"("Visible"=TRUE, "Scale.Maximum"=100.0 ("Scale.Range:Maximum")) -> ()  [unwired: 2 in, 2 out]
                n200 = property on="Test Ring" class="Ring (strict)"("Visible"=FALSE) -> ()  [unwired: 2 in, 2 out]
              }
            }
          }
        }
        n201 = property on="Progress" class="Clust (strict)"("Visible"=FALSE) -> ()  [unwired: 2 in, 2 out]
      }
      event "Test Name": Mouse Enter {
        # "Populate the ring with the list of tests"
        n202 = event-data() -> ()  [unwired: 1 in, 1 out]
        n203 = call <vilib>:"NT Read String Array.vi"("name"="TestMode/TestList" ("Name")) -> ("value"=w329:string[])  [unwired: 8 in, 2 out]
        n204 = Build Array (concatenate)("Select the test to run...", w329) -> (w328:string[])
        n205 = property on="Test Name" class="Ring (strict)"("Strings []"=w328) -> ()  [unwired: 2 in, 2 out]
      }
      event "Test Name": Value Change {
        w330 = FALSE ("Visible")
        # "Tell the robot the test name to run"
        n206 = event-data() -> ("NewVal"=w334:u16)  [unwired: 1 in]
        n207 = property on="Test Name" class="Ring (strict)"() -> ("Strings []"=w335:string[])  [unwired: 2 in, 2 out]
        n208 = local write "Progress"(T7 {"Test Progress"=0, "Test Progress Text"=""} ("Progress")) -> ()
        n209 = Index Array(array=w335, index=w334) -> (element=w333:string)
        n210 = call <vilib>:"NT Write String.vi"("value"=w333, "name"="TestMode/TestName" ("Name")) -> ()  [unwired: 9 in, 1 out]
        n211 = property on="Progress" class="Clust (strict)"("Visible"=TRUE) -> ()  [unwired: 2 in, 2 out]
        n212 = property on="Motor" class="Clust (strict)"("Visible"=w330) -> ()  [unwired: 2 in, 2 out]
        n213 = property on="Test Slider" class="Slide (strict)"("Visible"=w330) -> ()  [unwired: 2 in, 2 out]
        n214 = property on="On/Off" class="Bool (strict)"("Visible"=w330) -> ()  [unwired: 2 in, 2 out]
        n215 = property on="Rev/Fwd" class="Clust (strict)"("Visible"=w330) -> ()  [unwired: 2 in, 2 out]
        n216 = property on="Test Ring" class="Ring (strict)"("Visible"=w330) -> ()  [unwired: 2 in, 2 out]
      }
      event "Select Auto": Mouse Enter {
        # "Populate the combo box with the list of autonomous options"
        n217 = event-data() -> ()  [unwired: 1 in, 1 out]
        n218 = call <vilib>:"NT Read String Array.vi"("name"="Auto List" ("Name")) -> ("value"=w337:string[])  [unwired: 8 in, 2 out]
        n219 = property on="Select Auto" class="CmbBox"("Strings[]"=w337) -> ()  [unwired: 2 in, 2 out]
      }
      event "Select Auto": Value Change {
        # "User modified the Auto Selection. Write to NT variable so robot knows."
        n220 = event-data() -> ("NewVal"=w339:string)  [unwired: 1 in]
        n221 = call <vilib>:"NT Write String.vi"("value"=w339, "name"="Auto Selector" ("Name")) -> ()  [unwired: 9 in, 1 out]
      }
      event "CheckList": Double Click {
        # "Shift clears all"
        # "Update symbols on the listbox"
        n222 = event-data() -> ("PlatMods.Shift"=w341:bool, "Row"=w343:i32)  [unwired: 1 in]
        n223 = case shown="True" w341 {
          tunnel: w343 -> [w347 _]
          tunnel: 1 -> [w346 _]
          frame False {
            n224 = property on="CheckList" class="LstBox (strict)"() -> ("Item Symbols"=w345:i32[])  [unwired: 2 in, 2 out]
            n225 = Replace Array Subset(array=w345, new element=w346, index=w347) -> (w344:i32[])
            n226 = property on="CheckList" class="LstBox (strict)"("Item Symbols"=w344) -> ()  [unwired: 2 in, 2 out]
          }
          frame True {
            w348 = 0 ("Top Row")
            n227 = property on="CheckList" class="LstBox (strict)"() -> ("Number of Rows"=w350:u32)  [unwired: 2 in, 2 out]
            n228 = Initialize Array(0, w350) -> (w349:i32[])
            n229 = property on="CheckList" class="LstBox (strict)"("Top Row"=w348, "Value"=w348, "Item Symbols"=w349) -> ()  [unwired: 2 in, 2 out]
          }
        }
      }
      event "CheckList": Key Down {
        # "Update symbols on the listbox\nLeft and right keys check and uncheck"
        n230 = event-data() -> ("VKey"=w353:T23)  [unwired: 1 in]
        n231 = case shown="\"Left\", \"Right\"" w353 {
          selector: w353 -> [w358 _]
          tunnel: eventvkey."Left" ("VKey") -> [w356 _]
          frame "Left", "Right" {
            n232 = Equal?(x=w356, y=w358) -> (x = y?=w357:bool)
            n233 = Select(t=0, s=w357, f=1) -> (s? t:f=w359:i32)
            n234 = property on="CheckList" class="LstBox (strict)"() -> ("Item Symbols"=w362:i32[])  [unwired: 2 in, 2 out]
            n235 = Replace Array Subset(array=w362, new element=w359, index="CheckList") -> (w361:i32[])
            n236 = property on="CheckList" class="LstBox (strict)"("Item Symbols"=w361) -> ()  [unwired: 2 in, 2 out]
          }
          frame Default {
          }
        }
      }
      event "Motor.Enable": Value Change {
        # "When the test mode otor enable helper is set, update that\ntree row item's value"
        n237 = event-data() -> ("NewVal"=w367:bool)  [unwired: 1 in]
        n238 = Unbundle("Motor") -> ("Value"=w366:dbl)  [unwired: 1 out]
        n239 = Select(t=w366, s=w367, f=0.0) -> (s? t:f=w364:dbl)
        n240 = call <vilib>:"NT Write Number.vi"("value"=w364, "name"=w363) -> ()  [unwired: 9 in, 1 out]
      }
      event "Test Slider": Value Change {
        # "When the test mode slider helper is set, update that\ntree row item's value"
        n241 = event-data() -> ("NewVal"=w369:dbl)  [unwired: 1 in]
        n242 = call <vilib>:"NT Write Number.vi"("value"=w369, "name"=w370) -> ()  [unwired: 9 in, 1 out]
      }
      event "On/Off": Value Change {
        # "When the test mode on/off helper value is set, update that\ntree row item's value"
        n243 = event-data() -> ("NewVal"=w373:bool)  [unwired: 1 in]
        n244 = Boolean To (0,1)(Boolean=w373) -> (0, 1=w372:i16)
        n245 = call <vilib>:"NT Write Number.vi"("value"=w372, "name"=w371) -> ()  [unwired: 9 in, 1 out]
      }
      event "Rev/Fwd": Value Change {
        # "When the test mode helper value for relays is set, update that\ntree row item's value"
        n246 = event-data() -> ("NewVal.Forward"=w380:bool, "NewVal.Reverse"=w379:bool)  [unwired: 1 in]
        n247 = Boolean To (0,1)(Boolean=w380) -> (0, 1=w376:i16)
        n248 = Boolean To (0,1)(Boolean=w379) -> (0, 1=w378:i16)
        n249 = Negate(x=w378) -> (-x=w377:i16)
        n250 = Add(x=w376, y=w377) -> (x+y=w375:i16)
        n251 = call <vilib>:"NT Write Number.vi"("value"=w375, "name"=w374) -> ()  [unwired: 9 in, 1 out]
      }
      event "Test Ring": Value Change {
        # "When a test mode helper value is selected from the ring,\nset the tree item's variable to the string value"
        n252 = event-data() -> ("NewVal"=w383:u16)  [unwired: 1 in]
        n253 = property on="Test Ring" class="Ring (strict)"() -> ("Strings []"=w384:string[])  [unwired: 2 in, 2 out]
        n254 = Index Array(array=w384, index=w383) -> (element=w382:string)
        n255 = call <vilib>:"NT Write String.vi"("value"=w382, "name"=w381) -> ()  [unwired: 9 in, 1 out]
      }
      event "Rec Mode": Value Change {
        # "Update globals for recording mode and path to read log from.\nClear when logging and let NetworkTables set path for vision to\nuse."
        n256 = event-data() -> ("NewVal"=w393:enum32{"Stop", "Record", "Playback"})  [unwired: 1 in]
        n257 = global write "WPI_DashboardLogging Global.vi" "Logging Filename"(path "") -> ()
        n258 = global write "WPI_DashboardLogging Global.vi" "Recording"(w393) -> ()
        n259 = case shown="\"Playback\"" w393 {
          tunnel: w392 -> [_ w395 w403]
          tunnel: [_ _ w402] -> w390
          tunnel: [_ _ w401] -> _
          tunnel: w388 -> [_ _ w399]
          tunnel: cluster{i32, i32} {-250, 170} -> [_ _ w398]
          tunnel: [_ _ T24 {"Image Size"=TRUE, "Image Type"=TRUE, "Pixel Value"=TRUE, "ROI Information"=TRUE, "Zoom Factor"=FALSE} ("Image Information Shown:All Elements")] -> w385
          tunnel: [_ _ TRUE ("Zoom Factor")] -> w386
          frame Default {
          }
          frame "Stop", "Record" {
            # "Place Window too"
            n260 = invoke class="VI" method="FP.Close"(reference=w395) -> (reference out=w394:refnum<vi>)  [unwired: 2 in, 2 out]
            n261 = invoke class="VI" method="Abort VI"(reference=w394) -> ()  [unwired: 2 in, 3 out]
          }
          frame "Playback" {
            n262 = call "Open Playback Panel.vi"("Offset"=w398, "DB VI Ref"=w399, "Playback in"=w403) -> ("Playback out"=w400:refnum<vi>)  [unwired: 8 in]
            n263 = register-events(w400) -> (reference out=w402:refnum<event-registration>, error out=w401:errorcluster)  [unwired: 2 in]
          }
        }
        n264 = property on="Camera Image Right" class="ImageControl"("Image Information Shown"=w385, "Image Information Visible"=w386) -> ()  [unwired: 2 in, 2 out]
        n265 = property on="Camera Image" class="ImageControl"("Image Information Shown"=w385, "Image Information Visible"=w386) -> ()  [unwired: 2 in, 2 out]
        n266 = call <vilib>:"WPI_DashboardNT Log FieldName Cache.vi"("Operation"=enum16{"Lookup/Add", "Index", "Clear"}."Clear") -> ()  [unwired: 8 in, 3 out]
      }
      event Panel Close {
        w404 = enum32{"Stop", "Record", "Playback"}."Stop" ("Rec Mode")
        # "Playback window has been closed, abort"
        n267 = event-data() -> ()  [unwired: 1 in, 4 out]
        n268 = local write "Rec Mode"(w404) -> ()
        n269 = global write "WPI_DashboardLogging Global.vi" "Recording"(w404) -> ()
      }
      event Panel Close {
        # "Abort playback window and ourself"
        n270 = event-data() -> ()  [unwired: 1 in, 4 out]
        n271 = invoke class="VI" method="FP.Close"(reference=w407) -> (reference out=w406:refnum<vi>)  [unwired: 2 in, 2 out]
        n272 = invoke class="VI" method="Abort VI"(reference=w406) -> (error out=w405:errorcluster)  [unwired: 2 in, 2 out]
        n273 = invoke class="VI" method="Abort VI"(error in=w405) -> ()  [unwired: 2 in, 3 out]
      }
      event "Tree": Double Click {
        n274 = event-data() -> ("PlatMods"=w413:T26, "Tag"=w410:string)  [unwired: 1 in]
        n275 = Unbundle(w413) -> ("Shift"=w412:bool)  [unwired: 4 out]
        n276 = String Subset(string=w410, length (rest)=1 ("length (rest)")) -> (substring=w409:string)  [unwired: 1 in]
        n277 = Not(x=w412) -> (.not. x?=w411:bool)
        n278 = case shown="\"/\"" w409 {
          tunnel: w410 -> [_ w415]
          tunnel: w411 -> [_ w414]
          frame Default {
          }
          frame "/" {
            n279 = call <vilib>:"NT Update Persistence.vi"("Persistence"=w414, "Name"=w415) -> ()  [unwired: 9 in, 1 out]
          }
        }
      }
    }
  }
  n280 = while {
    tunnel: w54 -> [w417]
    i -> [w420]
    stop <- FALSE stop-if-true
    n281 = Wait (ms)(milliseconds to wait=u32 100) -> ()  [unwired: 1 out]
    n282 = case shown="\"Playback\"" "Rec Mode" {
      tunnel: w420 -> [_ _ w435]
      tunnel: [u32 2829099 ("Base Color") u32 11141120 ("Target Color") w424] -> w416
      frame "Stop", Default {
        # "Reset the color, extra updates don't cost much"
      }
      frame "Record" {
      }
      frame "Playback" {
        # "Playback"
        n283 = Quotient & Remainder(x=w435, y=u32 50 ("milliseconds to wait")) -> (x-y*floor(x/y)=w431:u32)  [unwired: 1 out]
        n284 = Divide(x=w431, y=u32 50 ("milliseconds to wait")) -> (x/y=w428:dbl)
        n285 = Multiply(x=6.283185307179586, y=w428) -> (x*y=w433:dbl)
        n286 = Sine(x=w433) -> (sin(x)=w432:dbl)
        n287 = Absolute Value(x=w432) -> (abs(x)=w425:dbl)
        n288 = call "Interpolate RGB Color.vi"("Proportion"=w425, "Target Color"=u32 30976, "Base Color"=u32 2829099) -> ("Result Color"=w424:u32)  [unwired: 8 in]
      }
    }
    n289 = property class="Pane"(reference=w417, "PaneColor"=w416) -> ()  [unwired: 1 in, 2 out]
  }
  n290 = local write "Dashboard Tab"(T2."Drive" ("Dashboard Tab")) -> ()
  n291 = property on="On/Off" class="Bool (strict)"("Visible"=w26) -> ()  [unwired: 2 in, 2 out]
  n292 = property on="Motor" class="Clust (strict)"("Visible"=w26) -> ()  [unwired: 2 in, 2 out]
  n293 = property on="Progress" class="Clust (strict)"("Visible"=w26) -> ()  [unwired: 2 in, 2 out]
  n294 = property on="Test Ring" class="Ring (strict)"("Visible"=w26) -> ()  [unwired: 2 in, 2 out]
  n295 = property on="Rev/Fwd" class="Clust (strict)"("Visible"=w26) -> ()  [unwired: 2 in, 2 out]
  n296 = while {
    tunnel: u16 1741 ("timeout ms (25000)") -> [w437]
    stop <- FALSE stop-if-true
    n297 = TCP Create Listener(10:w437) -> (0:w436:errorcluster, 3:w438:refnum<k5>)  [unwired: 4 in, 1 out]
    n298 = case shown="No Error" w436 {
      selector: w436 -> [w440 _]
      tunnel: w438 -> [w441 _]
      frame No Error {
        n299 = while {
          tunnel: w441 -> [w444]
          tunnel: w440 -> [w443]
          stop <- FALSE stop-if-true
          n300 = TCP Wait On Listener(8:w443, 11:w444) -> (0:w445:errorcluster, 4:w446:refnum<k5>)  [unwired: 2 in, 3 out]
          n301 = local write "TCP"(w446) -> ()
          n302 = case shown="Error" w445 {
            frame No Error {
            }
            frame Error {
              n303 = Wait (ms)(milliseconds to wait=u32 1000) -> ()  [unwired: 1 out]
            }
          }
        }
      }
      frame Error {
        n304 = Wait (ms)(milliseconds to wait=u32 1000) -> ()  [unwired: 1 out]
      }
    }
  }
  n305 = global write "WPI_DashboardLogging Global.vi" "Recording"(w49) -> ()
  n306 = local write "Rec Mode"(w49) -> ()
  n307 = call <vilib>:"NT Write String.vi"("value"="Select Auto", "name"="Auto Selector" ("Name")) -> ()  [unwired: 9 in, 1 out]
